vi "checksum.vi"(10 "chksum":i32, 11 "data":cluster{"engine":i32, "shaft":i32}) -> (0 "x = y?":bool, 3 "x-y*floor(x/y)":u8)   [LabVIEW 2013]
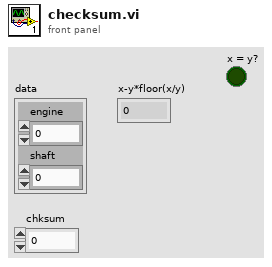
[diagram p1: front panel]
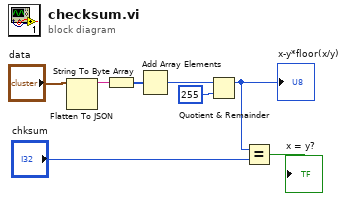
[diagram p0: block diagram]
diagram:
  n1 = Flatten To JSON(anything="data") -> (JSON string=w1:string)  [unwired: 2 in, 1 out]
  n2 = String To Byte Array(string=w1) -> (unsigned byte array=w2:u8[])
  n3 = Add Array Elements(numeric array=w2) -> (sum=w3:u8)
  n4 = Quotient & Remainder(x=w3, y=u8 255) -> (x-y*floor(x/y)=w6:u8)  [unwired: 1 out]
  "x-y*floor(x/y)" <- w6
  n5 = Equal?(x=w6, y="chksum") -> (x = y?=→"x = y?":bool)
